vi "Abort.Wait on Abort or Timeout.vi"(7 "Abort Notifier Name":string="Abort", 11 "Timeout ms (-1)":i32=-1) -> (2 "Timeout":bool, 3 "Abort":bool)   [LabVIEW 2024]
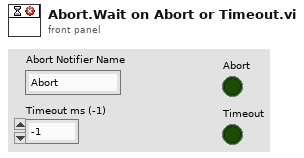
[diagram p1: front panel]
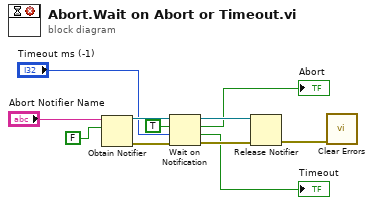
[diagram p0: block diagram]
diagram:
  n1 = Obtain Notifier(name (unnamed)="Abort Notifier Name", notification data type=FALSE) -> (notifier out=w9:refnum<notifier>, error out=w8:errorcluster)  [unwired: 2 in, 1 out]
  n2 = Wait on Notification(notifier=w9, ignore previous (F)=TRUE, timeout in ms (-1)="Timeout ms (-1)", error in (no error)=w8) -> (notifier out=w6:refnum<notifier>, notification=→"Abort":bool, timed out?=→"Timeout":bool, error out=w7:errorcluster)
  n3 = Release Notifier(notifier=w6, error in (no error)=w7) -> (error out=w4:errorcluster)  [unwired: 1 in, 2 out]
  n4 = call <vilib>:"Clear Errors.vi"("error in (no error)"=w4) -> ()  [unwired: 5 in, 2 out]
